vi "GetCurrentAvg.vi"(11 "RobotDriveDevRef":T1={"DevStatus"={"status"=FALSE, "code"=0, "source"=""}, "Motors[]"=[], "Square Inputs"=FALSE, "Max Output"=1.0, "Isochronous"=FALSE}) -> (3 "Current Avg":dbl)   [LabVIEW 2011]
uses:
  <vilib>/Rock Robotics/WPI/RobotDrive/WPI_RobotDriveDevRef.ctl
  <vilib>/Rock Robotics/WPI/MotorControl/WPI_MotorControlDeviceRef.ctl
  <vilib>/Rock Robotics/SystemInterfaces/Typedef/FPGA_TypedefDigitalModule.ctl
  <vilib>/Rock Robotics/SystemInterfaces/DIO/FPGA_DIOPWMChannel.ctl
  <vilib>/Rock Robotics/WPI/PWM/WPI_PWMDeadband.ctl
  <vilib>/Rock Robotics/WPI/CAN/Jaguar/SubVIs/WPI_CANJaguar_ControlMode.ctl
  <vilib>/Rock Robotics/WPI/PWM/WPI_PWMTransform_ConPane.ctl
  <vilib>/Rock Robotics/WPI/CAN/Jaguar/SubVIs/WPI_CANJaguar_StatusSelect.ctl
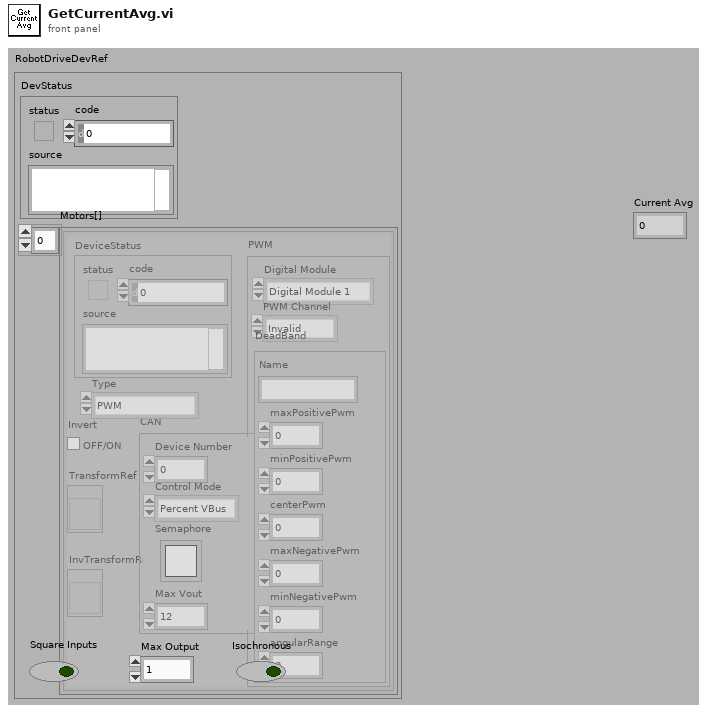
[diagram p1: front panel]
types:
  T1 = typedef "WPI_RobotDriveDevRef.ctl" = cluster{"DevStatus":errorcluster, "Motors[]":T2[], "Square Inputs":bool, "Max Output":dbl, "Isochronous":bool}
  T2 = typedef "WPI_MotorControlDeviceRef.ctl" = cluster{"DeviceStatus":errorcluster, "Type":enum16{"PWM", "CAN"}, "PWM":cluster{"Digital Module":T3, "PWM Channel":T4, "DeadBand":T5}, "CAN":cluster{"Device Number":u8, "Control Mode":T6, "Semaphore":T7, "Max Vout":dbl}, "Invert":bool, "TransformRef":T8, "InvTransformRef":T8}
  T3 = typedef "FPGA_TypedefDigitalModule.ctl" = enum16{"Digital Module 1", "Digital Module 2"}
  T4 = typedef "FPGA_DIOPWMChannel.ctl" = enum8{"PWM 1", "PWM 2", "PWM 3", "PWM 4", "PWM 5", "PWM 6", "PWM 7", "PWM 8", "PWM 9", "PWM 10", "Invalid"}
  T5 = typedef "WPI_PWMDeadband.ctl" = cluster{"Name":string, "maxPositivePwm":i32, "minPositivePwm":i32, "centerPwm":i32, "maxNegativePwm":i32, "minNegativePwm":i32, "angularRange":u16}
  T6 = typedef "WPI_CANJaguar_ControlMode.ctl" = enum8{"Percent VBus", "Current", "Speed", "Position", "Voltage"}
  T7 = typedef "Semaphore RefNum" = refnum<k1>
  T8 = typedef "WPI_PWMTransform_ConPane.ctl" = refnum<vi>
  T9 = typedef "WPI_CANJaguar_StatusSelect.ctl" = enum16{"Output Percent VBus", "Output Voltage", "Bus Voltage", "Current", "Temperature", "Position", "Speed", "Limit Switches", "Faults", "Fault Counters", "Power Cycle"}
  T10 = typedef "WPI_CANJaguar_Status.ctl" = cluster{"Output Percent VBus":dbl, "Output Voltage":dbl, "Bus Voltage":dbl, "Current":dbl, "Temperature":dbl, "Position":dbl, "Speed":dbl, "Limits":cluster{"Forward Limit":bool, "Reverse Limit":bool, "Forward Soft Limit":bool, "Reverse Soft Limit":bool, "Sticky Forward Limit":bool, "Sticky Reverse Limit":bool, "Sticky Forward Soft Limit":bool, "Sticky Reverse Soft Limit":bool}, "Faults":cluster{"Current Fault":bool, "Temperature Fault":bool, "Bus Voltage Fault":bool, "Gate Driver Fault":bool, "Comm Fault":bool}, "Fault Counters":cluster{"Current Faults":u8, "Temperature Faults":u8, "Bus Voltage Faults":u8, "Gate Driver Faults":u8, "Comm Faults":u8, "CAN Status":u8, "CAN RX Errors":u8, "CAN TX Errors":u8}, "Power Cycle":bool}
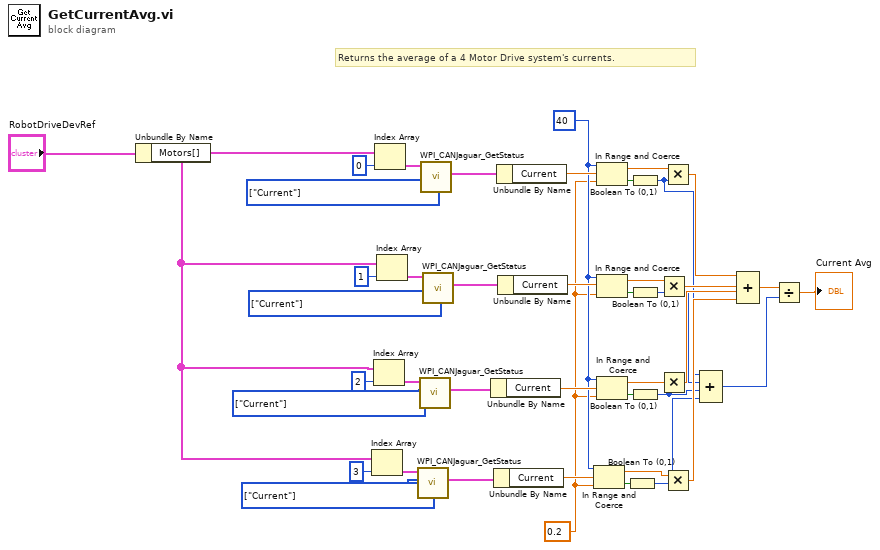
[diagram p0: block diagram]
diagram:
  w13 = 0.2
  w14 = 40
  w34 = T9[] [enum."Current"] items=["Output Percent VBus", "Output Voltage", "Bus Voltage", "Current", "Temperature", "Position", "Speed", "Limit Switches", "Faults", "Fault Counters", "Power Cycle"] ("Status Select")
  w33 = T9[] [enum."Current"] items=["Output Percent VBus", "Output Voltage", "Bus Voltage", "Current", "Temperature", "Position", "Speed", "Limit Switches", "Faults", "Fault Counters", "Power Cycle"] ("Status Select")
  w32 = T9[] [enum."Current"] items=["Output Percent VBus", "Output Voltage", "Bus Voltage", "Current", "Temperature", "Position", "Speed", "Limit Switches", "Faults", "Fault Counters", "Power Cycle"] ("Status Select")
  w31 = T9[] [enum."Current"] items=["Output Percent VBus", "Output Voltage", "Bus Voltage", "Current", "Temperature", "Position", "Speed", "Limit Switches", "Faults", "Fault Counters", "Power Cycle"] ("Status Select")
  # "Returns the average of a 4 Motor Drive system's currents."
  n1 = Unbundle By Name("RobotDriveDevRef") -> ("Motors[]"=w35:T2[])
  n2 = Index Array(array=w35, index=3) -> (element=w37:T2)
  n3 = Index Array(array=w35, index=2) -> (element=w38:T2)
  n4 = Index Array(array=w35, index=0) -> (element=w42:T2)
  n5 = Index Array(array=w35, index=1) -> (element=w41:T2)
  n6 = call <vilib>:"WPI_CANJaguar_GetStatus.vi"("Status Select"=w34, "CAN Jaguar Ref"=w37) -> ("Status"=w27:T10)  [unwired: 2 in, 7 out]
  n7 = call <vilib>:"WPI_CANJaguar_GetStatus.vi"("Status Select"=w33, "CAN Jaguar Ref"=w38) -> ("Status"=w28:T10)  [unwired: 2 in, 7 out]
  n8 = call <vilib>:"WPI_CANJaguar_GetStatus.vi"("Status Select"=w31, "CAN Jaguar Ref"=w42) -> ("Status"=w30:T10)  [unwired: 2 in, 7 out]
  n9 = call <vilib>:"WPI_CANJaguar_GetStatus.vi"("Status Select"=w32, "CAN Jaguar Ref"=w41) -> ("Status"=w29:T10)  [unwired: 2 in, 7 out]
  n10 = Unbundle By Name(w28) -> ("Current"=w16:dbl)
  n11 = Unbundle By Name(w27) -> ("Current"=w15:dbl)
  n12 = Unbundle By Name(w30) -> ("Current"=w17:dbl)
  n13 = Unbundle By Name(w29) -> ("Current"=w18:dbl)
  n14 = In Range and Coerce(upper limit=w14, x=w15, lower limit=w13) -> (coerced(x)=w8:dbl, In Range?=w19:bool)
  n15 = In Range and Coerce(upper limit=w14, x=w17, lower limit=w13) -> (coerced(x)=w9:dbl, In Range?=w22:bool)
  n16 = In Range and Coerce(upper limit=w14, x=w18, lower limit=w13) -> (coerced(x)=w10:dbl, In Range?=w21:bool)
  n17 = In Range and Coerce(upper limit=w14, x=w16, lower limit=w13) -> (coerced(x)=w11:dbl, In Range?=w20:bool)
  n18 = Boolean To (0,1)(Boolean=w19) -> (0, 1=w1:i16)
  n19 = Boolean To (0,1)(Boolean=w22) -> (0, 1=w3:i16)
  n20 = Boolean To (0,1)(Boolean=w21) -> (0, 1=w4:i16)
  n21 = Boolean To (0,1)(Boolean=w20) -> (0, 1=w2:i16)
  n22 = Multiply(x=w10, y=w4) -> (x*y=w12:dbl)
  n23 = Multiply(x=w11, y=w2) -> (x*y=w7:dbl)
  n24 = Multiply(x=w9, y=w3) -> (x*y=w5:dbl)
  n25 = Multiply(x=w8, y=w1) -> (x*y=w6:dbl)
  n26 = Compound Arithmetic op=ADD(w3, w4, w2, w1) -> (w24:i16)
  n27 = Compound Arithmetic op=ADD(w5, w12, w7, w6) -> (w25:dbl)
  n28 = Divide(x=w25, y=w24) -> (x/y=→"Current Avg":dbl)
